vi "acquire_image_pixelfly.vi"(3 "error in":errorcluster, 4 "Acquitsition Settings":T2, 5 "Control Reference Cluster Input":T1) -> (0 "error out":errorcluster, 1 "Buffer status":T3, 2 "Output array":dbl[][](array[numeric]) format="%.2f")   [LabVIEW 2016]
doc: "Take a single PixelFly exposure and display the result as an intensity graph.This VI illustrates the basics of taking an exposure with the PixelFly camera. Use Ctrl-H to get help on any of the controls\n\nCopyright 2001, The Cooke Corporation."
uses:
  Controls/PixelFly/PixelFly Buffer Status.ctl
  Controls/PixelFly/Acquisition Settings.ctl
panel:
  in  "Boolean\nPrototyple":bool
  # "Take a single PixelFly exposure and display the result as an intensity graph."
  # "This VI illustrates the basics of taking an exposure with the PixelFly camera. Use Ctrl-H to get help on any of the controls\n\nCopyright 2001, The Cooke Corporation."
  # "Note that the image is inverted. The image reads out from top to bottom, but intensity graph plots bottom to top"
  # "Status flags"
  # "Buffer errors"
  # "Memory usage"
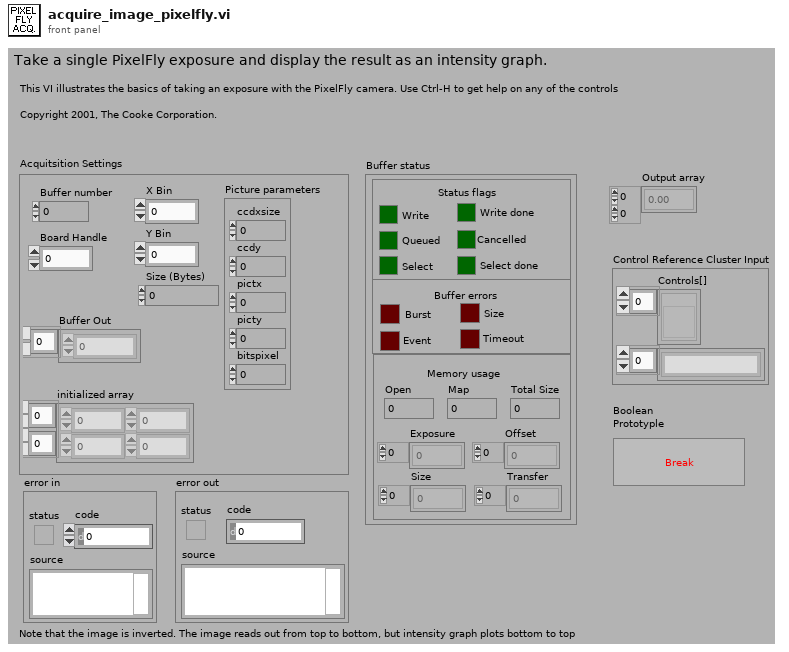
[diagram p1: front panel]
types:
  T1 = cluster{"Controls[]":refnum<vi>[], "Control Names":string[]}
  T2 = typedef "Acquisition Settings.ctl" = cluster{"Buffer number":i32, "Size (Bytes)":i32, "initialized array":u16[][], "X Bin":i32, "Y Bin":i32, "Board Handle":u32, "Picture parameters":cluster{"ccdxsize":i32, "ccdy":i32, "pictx":i32, "picty":i32, "bitspixel":i32}, "Buffer Out":u16[]}
  T3 = typedef "PixelFly Buffer Status.ctl" = cluster{"Write":bool, "Write done":bool, "Queued":bool, "Cancelled":bool, "Select":bool, "Select done":bool, "Burst":bool, "Size":bool, "Event":bool, "Timeout":bool, "Open":i32, "Map":i32, "Exposure":i32[], "Offset":i32[], "Size":i32[], "Transfer":i32[], "Total Size":i32}
  T4 = enum8{"Enabled", "Disabled", "Disabled and Grayed Out"}
  T5 = cluster{"ccdxsize":i32, "ccdy":i32, "pictx":i32, "picty":i32, "bitspixel":i32}
  T6 = cluster{"Write":bool, "Write done":bool, "Queued":bool, "Cancelled":bool, "Select":bool, "Select done":bool, "Burst":bool, "Size":bool, "Event":bool, "Timeout":bool, "Open":i32, "Map":i32, "Exposure":i32[], "Offset":i32[], "Size":i32[], "Transfer":i32[], "Total Size":i32}
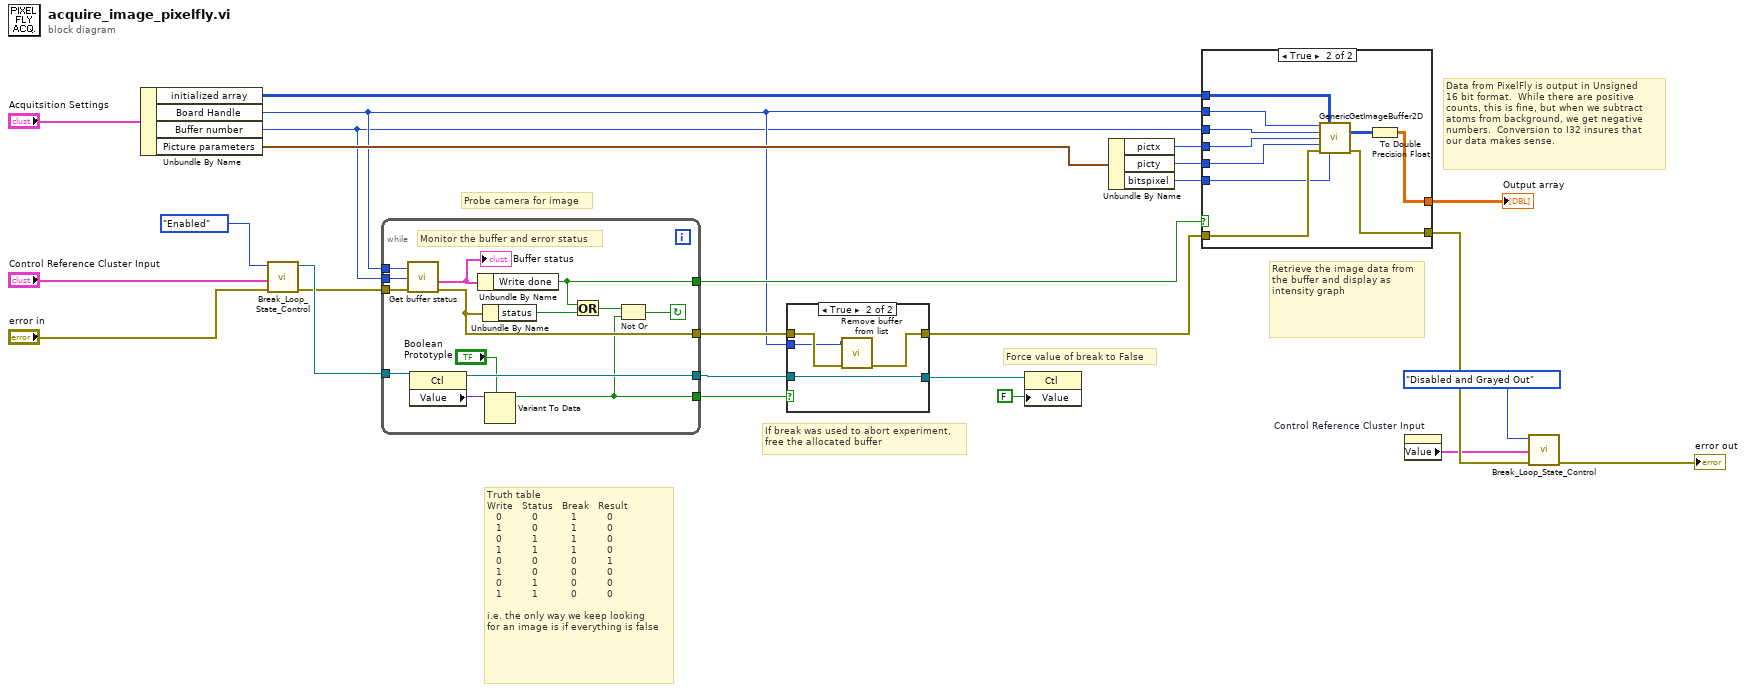
[diagram p0: block diagram]
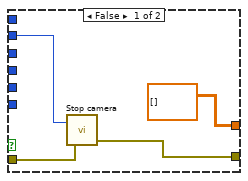
[diagram p3: hidden frame]
diagram:
  # "Force value of break to False"
  # "If break was used to abort experiment,\nfree the allocated buffer"
  # "Probe camera for image"
  # "Data from PixelFly is output in Unsigned\n16 bit format.  While there are positive\ncounts, this is fine, but when we subtract \natoms from background, we get negative\nnumbers.  Conversion to I32 insures that\nour data makes sense."
  # "Retrieve the image data from the buffer and display as intensity graph"
  # "Truth table\nWrite   Status   Break   Result\n   0          0           1          0\n   1          0           1          0\n   0          1           1          0\n   1          1           1          0\n   0          0           0          1\n   1          0           0          0\n   0          1           0          0\n   1          1           0          0\n\ni.e. the only way we keep looking\nfor an image is if everything is false"
  n1 = Unbundle By Name("Acquitsition Settings") -> ("initialized array"=w12:u16[][], "Board Handle"=w5:u32, "Buffer number"=w2:i32, "Picture parameters"=w16:T5)
  n2 = call "Break_Loop_State_Control.vi"("Error In"="error in", "Control Reference Cluster Input"="Control Reference Cluster Input", "Control State In"=T4."Enabled") -> ("error out"=w11:errorcluster, "Break Loop RefNum"=w21:refnum<vi>)  [unwired: 7 in]
  n3 = while {
    tunnel: w11 -> [w37]
    tunnel: w2 -> [w38]
    tunnel: w5 -> [w39]
    tunnel: [w34] -> w9
    tunnel: w21 -> [w33]
    tunnel: [w29] -> w4
    tunnel: [w27] -> w17
    tunnel: [w26] -> w7
    stop <- w31 continue-if-true
    # "Monitor the buffer and error status"
    n4 = call "Get buffer status.vi"("error in (no error)"=w37, "Buffer request"=w38, "Handle in"=w39) -> ("error out"=w34:errorcluster, "Buffer status"=w36:T6)  [unwired: 1 in, 2 out]
    "Buffer status" <- w36
    n5 = property class="Ctl"(reference=w33) -> (reference out=w29:refnum<vi>, "Value"=w32:variant)  [unwired: 1 in, 1 out]
    n6 = Unbundle By Name(w36) -> ("Write done"=w27:bool)
    n7 = Unbundle By Name(w34) -> ("status"=w35:bool)
    n8 = Variant To Data(type="Boolean\nPrototyple", Variant=w32) -> (data=w26:bool)  [unwired: 1 in, 1 out]
    n9 = Or(x=w27, y=w35) -> (x .or. y?=w30:bool)
    n10 = Not Or(1:w26, 2:w30) -> (0:w31:bool)
  }
  n11 = case shown="True" w7 {
    tunnel: w9 -> [w41 w44]
    tunnel: [w41 w43] -> w6
    tunnel: w5 -> [_ w42]
    tunnel: [w40 w45] -> w3
    tunnel: w4 -> [w40 w45]
    frame False {
    }
    frame True {
      n12 = call "Remove buffer from list.vi"("error in (no error)"=w44, "Handle in"=w42) -> ("error out"=w43:errorcluster)  [unwired: 4 in, 1 out]
    }
  }
  n13 = property class="Ctl"(reference=w3, "Value"=FALSE) -> ()  [unwired: 1 in, 2 out]
  n14 = Unbundle By Name(w16) -> ("pictx"=w13:i32, "picty"=w14:i32, "bitspixel"=w15:i32)
  n15 = case shown="True" w17 {
    tunnel: w2 -> [_ w55]
    tunnel: w6 -> [w49 w59]
    tunnel: [w48 w58] -> w20
    tunnel: w5 -> [w47 w57]
    tunnel: w12 -> [_ w56]
    tunnel: w15 -> [_ w54]
    tunnel: w14 -> [_ w53]
    tunnel: w13 -> [_ w52]
    tunnel: [dbl[][] [] w50] -> w1
    frame False {
      n16 = call "Stop camera.vi"("Handle in"=w47, "error in (no error)"=w49) -> ("error out"=w48:errorcluster)  [unwired: 2 out]
    }
    frame True {
      n17 = call "GenericGetImageBuffer2D.vi"("ph"=w57, "BuffIn"=w56, "BuffNr"=w55, "XRes"=w52, "YXRes"=w53, "error in (no error)"=w59, "BitRes"=w54) -> ("BuffOut"=w51:u16[][], "error out"=w58:errorcluster)  [unwired: 5 in, 2 out]
      n18 = To Double Precision Float(number=w51) -> (double precision float=w50:dbl[][])
    }
  }
  "Output array" <- w1
  n19 = property on="Control Reference Cluster Input" class="Clust (strict)"() -> ("Value"=w8:T1)  [unwired: 2 in, 2 out]
  n20 = call "Break_Loop_State_Control.vi"("Error In"=w20, "Control Reference Cluster Input"=w8, "Control State In"=T4."Disabled and Grayed Out") -> ("error out"=→"error out":errorcluster)  [unwired: 7 in, 1 out]
